vi "sv_Delay for Even-Angle Signal.vi"(0 "even-angle signals":cluster{"r0":dbl, "dr":dbl, "Y":dbl[]}[](array[cluster]), 2 "reset?":bool, 7 "even-angle position info":T1, 9 "delay [samples]":i32, 11 "error in (no error)":errorcluster, 13 "zero delay? (F)":bool) -> (4 "even-angle signals out":cluster{"r0":dbl, "dr":dbl, "Y":dbl[]}[](array[cluster]), 8 "even-angle position info out":T1, 15 "error out":errorcluster)   [LabVIEW 2017, in "SoundVib_ContSweptSine.lvlib"]
uses:
  <vilib>/addons/Sound and Vibration/svt_Continuous Swept Sine/SoundVib_ContSweptSine.lvlib
  <vilib>/addons/Sound and Vibration/Order Analysis/Misc/OAT Position Info.ctl
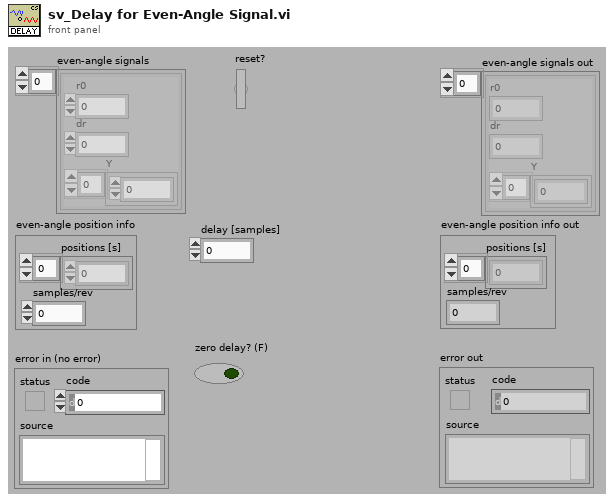
[diagram p1: front panel]
types:
  T1 = typedef "OAT Position Info.ctl" = cluster{"positions [s]":dbl[], "samples/rev":dbl}
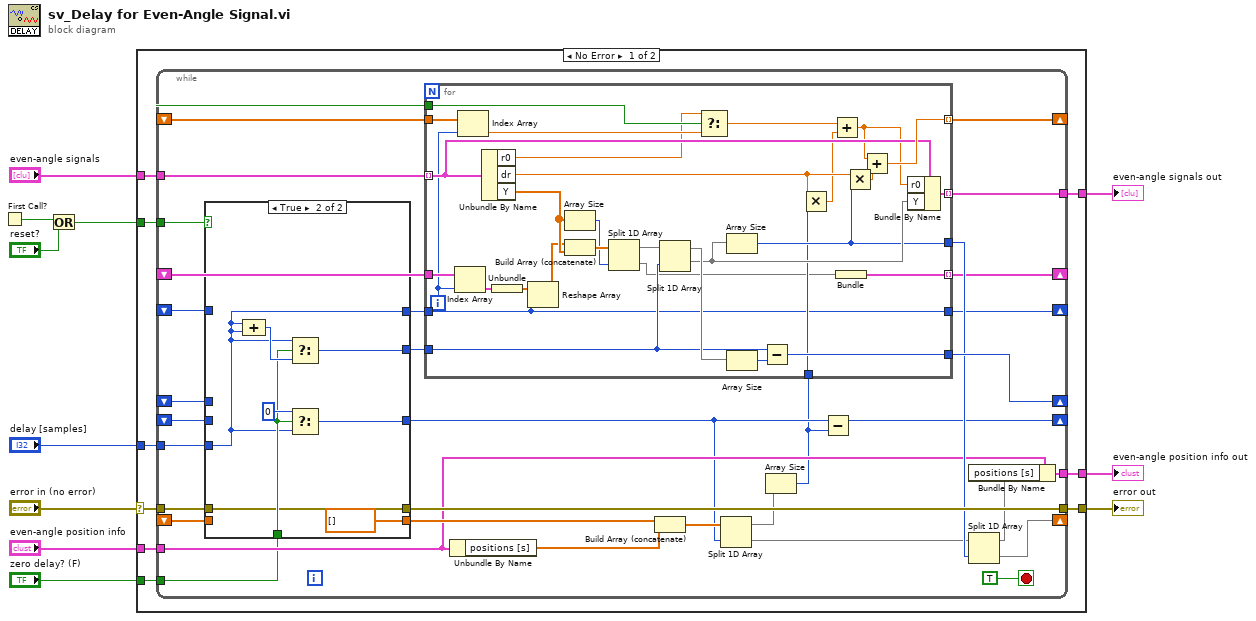
[diagram p0: block diagram]
diagram:
  n1 = First Call?() -> (First Call?: T/F=w11:bool)
  n2 = Or(x=w11, y="reset?") -> (x .or. y?=w9:bool)
  n3 = case shown="No Error" "error in (no error)" {
    selector: "error in (no error)" -> [w17 w100]
    tunnel: w9 -> [w20 _]
    tunnel: "even-angle signals" -> [w19 w99]
    tunnel: [w18 w99] -> w7
    tunnel: [w16 w100] -> w5
    tunnel: "even-angle position info" -> [w15 w98]
    tunnel: [w14 w98] -> w3
    tunnel: "zero delay? (F)" -> [w13 _]
    tunnel: "delay [samples]" -> [w12 _]
    frame No Error {
      n4 = while {
        tunnel: w20 -> [w50]
        tunnel: w19 -> [w52]
        shift-right: [w51] -> _
        shift-left: _ -> [w46]
        shift-right: [w49] -> _
        shift-left: _ -> [w48]
        tunnel: [w47] -> w18
        tunnel: w17 -> [w45]
        tunnel: [w44] -> w16
        tunnel: w15 -> [w36]
        shift-right: [w41] -> _
        shift-left: _ -> [w40]
        tunnel: [w35] -> w14
        shift-right: [w31] -> _
        shift-left: _ -> [w30]
        tunnel: w13 -> [w26]
        tunnel: w12 -> [w27]
        shift-right: [w25] -> _
        shift-left: _ -> [w24]
        shift-right: [w21] -> _
        shift-left: _ -> [w23]
        stop <- TRUE stop-if-true
        n5 = case shown="True" w50 {
          tunnel: w46 -> [w86 _]
          tunnel: w45 -> [w89 w92]
          tunnel: [w89 w92] -> w44
          tunnel: w40 -> [w88 _]
          tunnel: [w88 dbl[] []] -> w38
          tunnel: [w87 w93] -> w34
          tunnel: w30 -> [w87 _]
          tunnel: w26 -> [_ w94]
          tunnel: [w86 w91] -> w29
          tunnel: w27 -> [_ w90]
          tunnel: w23 -> [w85 _]
          tunnel: [w85 w90] -> w22
          frame False {
          }
          frame True {
            n6 = Compound Arithmetic op=ADD(w90, w90) -> (w96:i32)
            n7 = Select(t=w90, s=w94, f=w96) -> (s? t:f=w91:i32)
            n8 = Select(t=0, s=w94, f=w90) -> (s? t:f=w93:i32)
          }
        }
        n9 = Unbundle By Name(w36) -> ("positions [s]"=w43:dbl[])
        n10 = Build Array (concatenate)(w38, w43) -> (w39:dbl[])
        n11 = Split 1D Array(array=w39, index=w34) -> (first subarray=w32:dbl[], second subarray=w33:dbl[])
        n12 = Array Size(array=w32) -> (size(s)=w28:i32)
        n13 = for {
          tunnel: w52 -> [w80] mode=indexing
          tunnel: [w84] -> w51
          tunnel: w50 -> [w78]
          tunnel: [w81] -> w49 mode=indexing
          tunnel: w48 -> [w77]
          tunnel: [w76] -> w47 mode=indexing
          tunnel: [w74] -> w42
          tunnel: w29 -> [w73]
          tunnel: w28 -> [w71]
          tunnel: [w60] -> w25 mode=indexing
          tunnel: w24 -> [w59]
          tunnel: w22 -> [w55]
          tunnel: [w55] -> w21
          i -> [w58]
          n14 = Index Array(array=w59, index=w58) -> (element=w57:cluster{dbl[]})
          n15 = Index Array(array=w77, index=w58) -> (element=w75:dbl)
          n16 = Unbundle By Name(w80) -> ("r0"=w68:dbl, "dr"=w70:dbl, "Y"=w63:dbl[])
          n17 = Unbundle(w57) -> (w56:dbl[])
          n18 = Reshape Array(w56, w55) -> (w54:dbl[])
          n19 = Array Size(array=w63) -> (size(s)=w64:i32)
          n20 = Build Array (concatenate)(w54, w63) -> (w65:dbl[])
          n21 = Split 1D Array(array=w65, index=w64) -> (first subarray=w62:dbl[], second subarray=w61:dbl[])
          n22 = Split 1D Array(array=w62, index=w73) -> (first subarray=w83:dbl[], second subarray=w79:dbl[])
          n23 = Select(t=w68, s=w78, f=w75) -> (s? t:f=w67:dbl)
          n24 = Array Size(array=w79) -> (size(s)=w74:i32)
          n25 = Array Size(array=w83) -> (size(s)=w72:i32)
          n26 = Subtract(x=w73, y=w72) -> (x-y=w84:i32)
          n27 = Multiply(x=w70, y=w71) -> (x*y=w69:dbl)
          n28 = Add(x=w67, y=w69) -> (x+y=w66:dbl)
          n29 = Bundle(w61) -> (w60:cluster{dbl[]})  [unwired: 1 in]
          n30 = Multiply(x=w70, y=w74) -> (x*y=w82:dbl)
          n31 = Add(x=w66, y=w82) -> (x+y=w81:dbl)
          n32 = Bundle By Name(cluster=w80, "r0"=w66, "Y"=w79) -> (w76:cluster{"r0":dbl, "dr":dbl, "Y":dbl[]})
        }
        n33 = Subtract(x=w34, y=w28) -> (x-y=w31:i32)
        n34 = Split 1D Array(array=w33, index=w42) -> (first subarray=w37:dbl[], second subarray=w41:dbl[])
        n35 = Bundle By Name(cluster=w36, "positions [s]"=w37) -> (w35:T1)
      }
    }
    frame Error {
    }
  }
  "even-angle signals out" <- w7
  "error out" <- w5
  "even-angle position info out" <- w3
